vi "Marvin.vi"() -> ()   [LabVIEW 2017]
uses:
  PCAN_Driver/ControlCAN.llb/CAN Channel.ctl
  PCAN_Driver/ControlCAN.llb/DevType.ctl
  PCAN_Driver/ControlCAN.llb/VCI_INIT_CONFIG.ctl
  PCAN_Driver/ControlCAN.llb/InitFlag.ctl
  PCAN_Driver/ControlCAN.llb/Fliter.ctl
  PCAN_Driver/ControlCAN.llb/Mode.ctl
  <vilib>/Utility/miscctls.llb/LVMinMaxIncTypeDef.ctl
  PCAN_Driver/ControlCAN.llb/VCI_CAN_OBJ.ctl
  PCAN_Driver/ControlCAN.lvlib
panel:
  in  "Help Button":bool
  in  "Clear Monitor":bool
  out "Array":u64[][](array[numeric]) format="%016x"
  out "Waveform Chart":dbl[](graph)
  out "Ambient Over temp":bool
  out "Ambient Sensor temp":bool
  out "Ambient Temperature":dbl
  in  "Motor Over Temp":bool
  in  "Speed control":bool
  out "Unit Adress":string
  in  "Serial Send":bool
  in  "Index":u16(ring) items=["1"=1, "2"=2, "3"=3]
  out "read buffer":string
  in  "SetGet":enum16{"Get", "Set"}(ring)
  in  "Function":T1(ring)
  in  "Value":dbl
  in  "Value 1/2":enum16{"1", "2"}(ring)
  out "Msg Count":u32
  in  "Param to Set":u16(ring) items=["EBAY 5F"=95, "AHU 3F"=63, "AHU 2F"=47]
  out "Unit Adress":u8
  out "Horizontal Progress Bar":i32(slide) min=0 max=48 scale=0.0..50.0
  in  "Set Param.":bool
  in  "Serial Monitor":bool caption="Graph Button"
  in  "Serial Com":bool
  in  "VISA resource name":refnum<visa-resource-name>="COM6"
  out "Serial Status":bool
  in  "Graph Button":bool
  in  "Refresh Button":bool
  out "Data Send":u64 format="%016x"
  in  "Motor Speed RPM":u16
  out "Under voltage/Over voltage":bool
  out "Speed error":bool
  out "Derated drive temp":bool
  out "Motor Over temperature":bool
  out "Commutation err":bool
  out "Motor Sensor temp Fauilre":bool
  out "Drive Over temperature":bool
  out "Drive Sensor temp Failure":bool
  out "Motor Phase Current RMS":dbl
  out "ECS State":u16
  out "Motor Speed RPM":dbl
  out "Motor Stator Temp.":dbl
  out "Power transistor Heat sink Temp.":dbl
  out "DC Current":dbl
  out "DC Voltage":dbl
  in  "Can Send":bool
  in  "Stop":bool
  out "Config_CANAT":T8 {"DevType" items=["USB-CAN"=3, "USB-CAN2"=4]; "CanIndex" items=["通道1", "通道2"]; "VCI_INIT_CONFIG"."Fliter" items=["接收所有类型"=3, "只接收标准帧"=4, "只接收扩展帧"=7]; "VCI_INIT_CONFIG"."Mode" items=["正常工作", "自测模式（环回）", "仅侦听模式"]; "VCI_INIT_CONFIG"."InitFlag" items=["使用Flash参数", "使用界面设置参数"]}
  in  "Channel 2":T3 caption="Channel" items=["Channel 1", "Channel 2"]
  out "CAN Status":bool
  # "ver 1.3"
  # "Marvin"
  # "REDLER TECHNOLOGIES LTD"
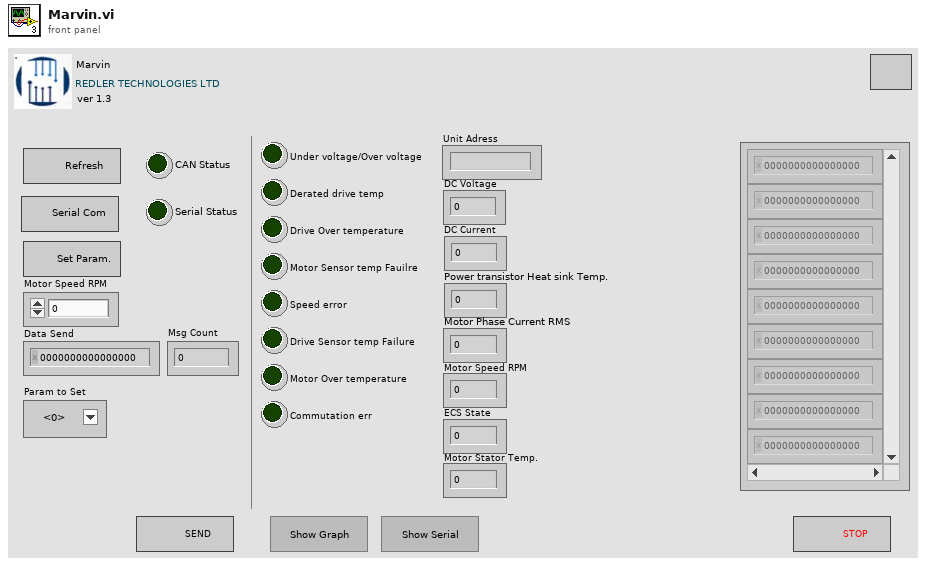
[diagram p1: front panel]
types:
  T1 = enum16{"Enable Conf. EP=1", "Serial Number", "Temperature", "Unit Adress", "Calibration", "Velocity", "Version"}
  T2 = typedef "ControlCAN.lvlib/DevType.ctl" = u32
  T3 = typedef "ControlCAN.lvlib/CAN Channel.ctl" = u32
  T4 = typedef "ControlCAN.lvlib/VCI_INIT_CONFIG.ctl" = cluster{"AccCode":u32, "AccMask":u32, "InitFlag":T5, "Fliter":T6, "Timing0":u8, "Timing1":u8, "Mode":T7}
  T5 = typedef "ControlCAN.lvlib/InitFlag.ctl" = u32
  T6 = typedef "ControlCAN.lvlib/Fliter.ctl" = u8
  T7 = typedef "ControlCAN.lvlib/Mode.ctl" = u8
  T8 = cluster{"DevType":T2, "DevIndex":u32, "CanIndex":T3, "VCI_INIT_CONFIG":T4}
  T9 = cluster{"ID":u32, "MSGTYPE":u8, "LEN":u8, "aDATA":u8[]}[]
  T10 = cluster{"ID":u32, "MSGTYPE":u8, "LEN":u8, "aDATA":u8[]}
  T11 = enum8{"Enabled", "Disabled", "Disabled and Grayed Out"}
  T12 = typedef "LVMinMaxIncTypeDef.ctl" = cluster{"Minimum":dbl, "Maximum":dbl, "Increment":dbl}
  T13 = enum32{"Invalid", "Standard", "Closed", "Hidden", "Minimized", "Maximized"}
  T14 = typedef "ControlCAN.lvlib/VCI_CAN_OBJ.ctl" = cluster{"ID":u32, "TimeStamp":u32, "TimeFlag":u8, "SendType":u8, "RemoteFlag":u8, "ExternFlag":u8, "DataLen":u8, "Data":u8[], "Reserved":u8[]}
  T15 = cluster{"Type":enum16{"接收", "发送"}, "Channel":T3, "Time":timestamp, "VCI_CAN_OBJ":T14}[]
  T16 = cluster{"Type":enum16{"接收", "发送"}, "Channel":T3, "Time":timestamp, "VCI_CAN_OBJ":T14}
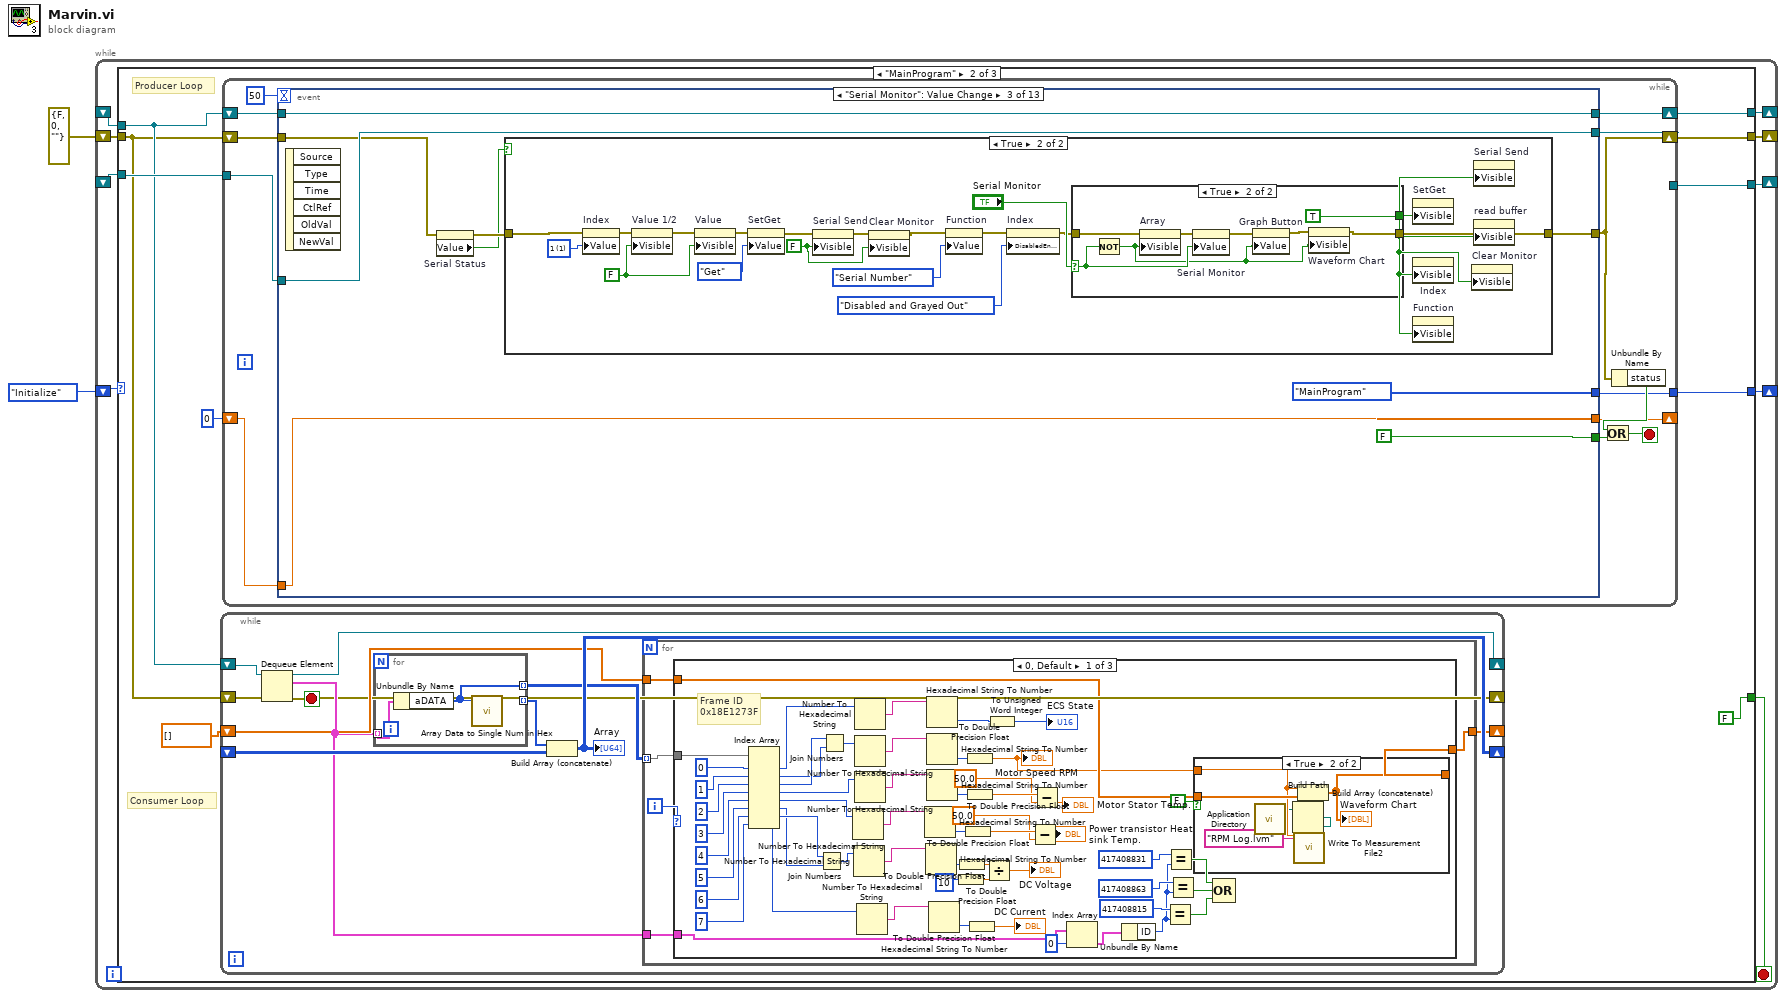
[diagram p0: block diagram]
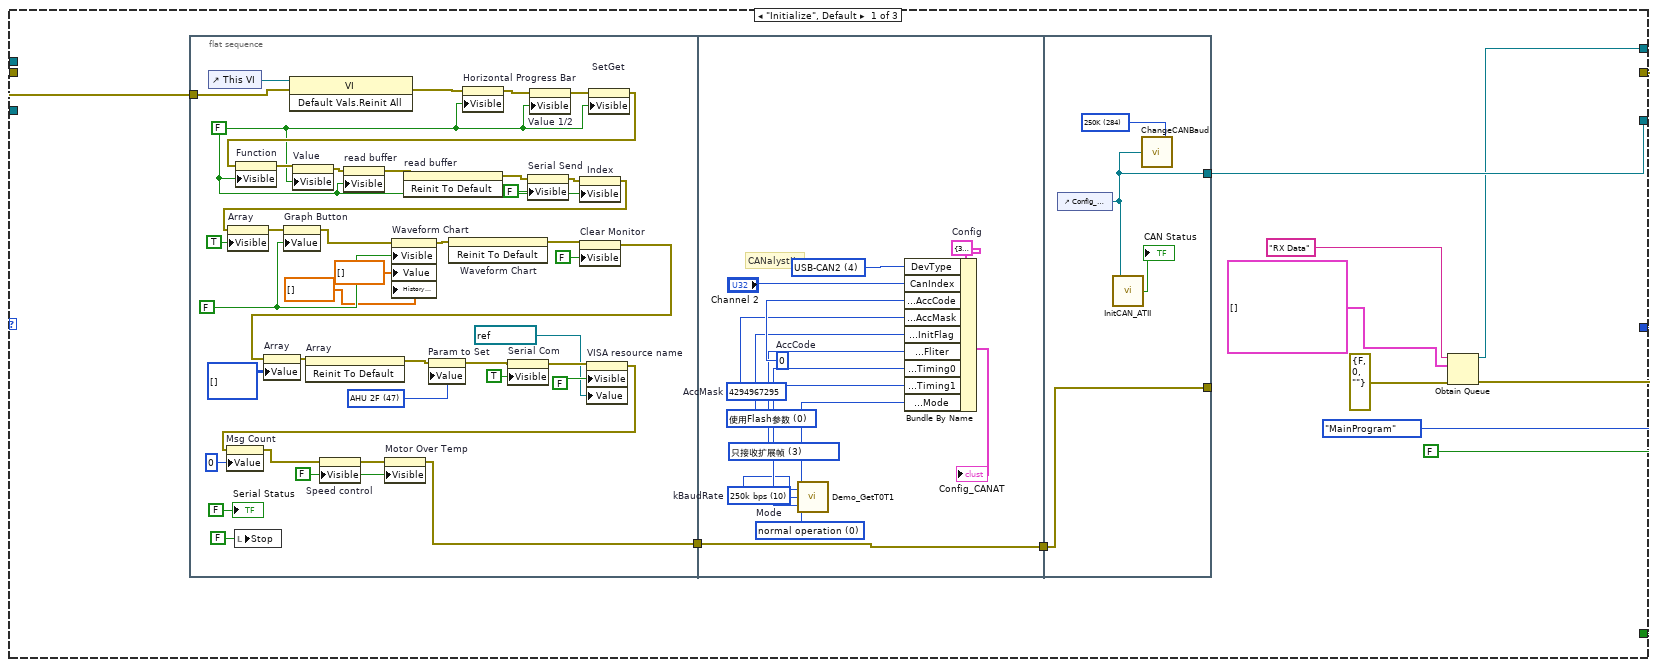
[diagram p2: hidden frame]
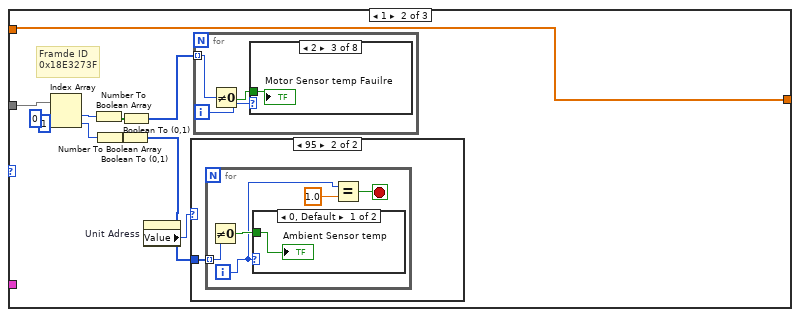
[diagram p4: hidden frame]
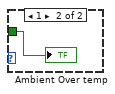
[diagram p6: hidden frame]
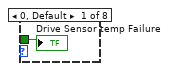
[diagram p7: hidden frame]
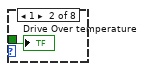
[diagram p8: hidden frame]
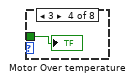
[diagram p9: hidden frame]
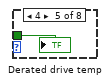
[diagram p10: hidden frame]
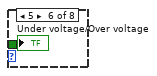
[diagram p11: hidden frame]
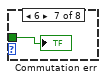
[diagram p12: hidden frame]
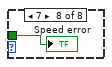
[diagram p13: hidden frame]
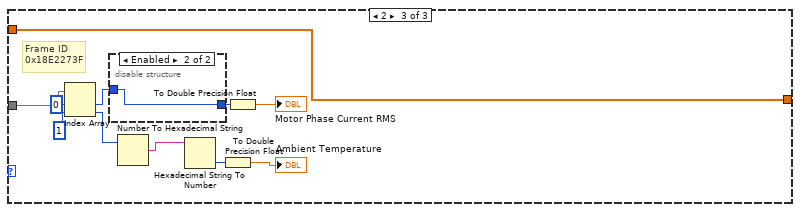
[diagram p14: hidden frame]
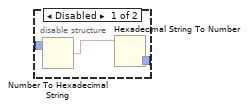
[diagram p15: hidden frame]
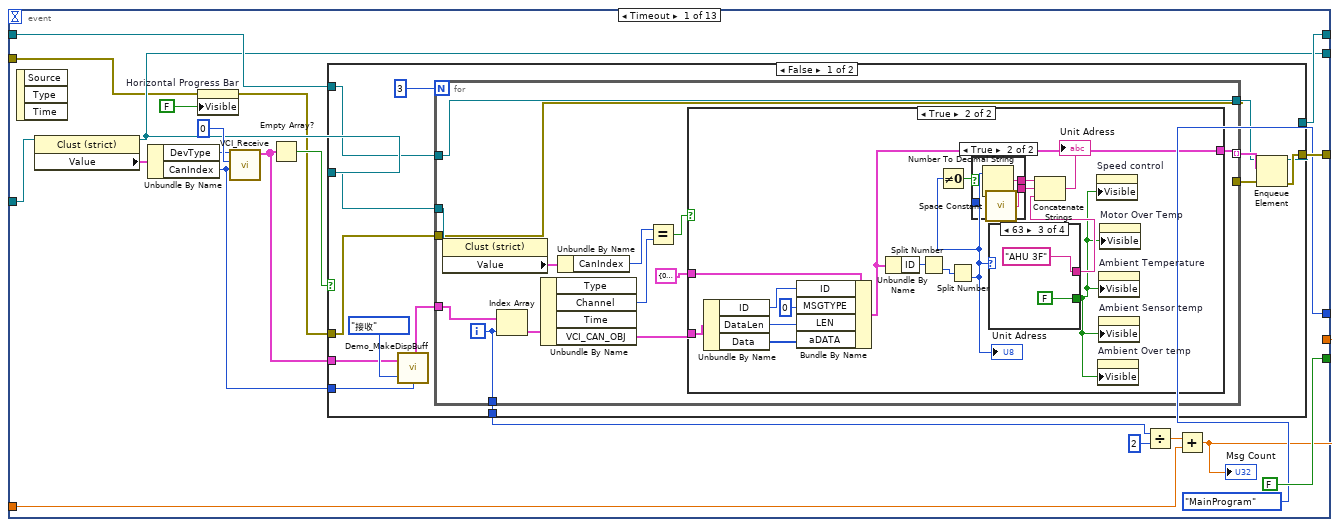
[diagram p16: hidden frame]
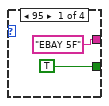
[diagram p19: hidden frame]
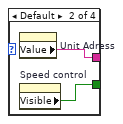
[diagram p20: hidden frame]
diagram:
  n1 = while {
    shift-right: [w6] -> _
    shift-left: enum16{"Stop", "MainProgram", "Initialize"}."Initialize" -> [w11]
    shift-right: [w10] -> _
    shift-left: _ -> [w9]
    shift-right: [w8] -> _
    shift-left: _ -> [w5]
    shift-right: [w7] -> _
    shift-left: errorcluster {"status"=FALSE, "code"=0, "source"=""} ("error out") -> [w4]
    stop <- w3 stop-if-true
    n2 = case shown="\"MainProgram\"" w11 {
      tunnel: [w22 w87 w865] -> w10
      tunnel: w9 -> [_ w90 w865]
      tunnel: [w18 w89 w866] -> w8
      tunnel: [w17 w88 w867] -> w7
      tunnel: [enum16{"Stop", "MainProgram", "Initialize"}."MainProgram" w86 enum16{"Stop", "MainProgram", "Initialize"}."Stop"] -> w6
      tunnel: w5 -> [_ w85 w866]
      tunnel: w4 -> [w15 w84 w868]
      tunnel: [FALSE ("Stop") FALSE ("Stop") w864] -> w3
      frame "Initialize", Default {
        n3 = flat-sequence {
          tunnel: w15 -> [w36]
          tunnel: [w32] -> w13
          tunnel: [w64] -> w14
          tunnel: w13 -> [w64]
          tunnel: [w78] -> w22
          tunnel: w14 -> [w77]
          tunnel: [w77] -> _
          frame #0 {
            w31 = FALSE ("Visible")
            w49 = u16 47 items=["EBAY 5F"=95, "AHU 3F"=63, "AHU 2F"=47] ("Param to Set")
            w26 = FALSE ("Visible")
            w55 = FALSE ("Graph Button")
            n4 = control-ref of="This VI"() -> (w63:refnum<vi>)
            n5 = local write "Stop"(FALSE ("Stop")) -> ()
            n6 = invoke class="VI" method="Default Vals.Reinit All"(reference=w63, error in=w36) -> (error out=w35:errorcluster)  [unwired: 1 in, 2 out]
            n7 = property on="Horizontal Progress Bar" class="Slide (strict)"(error in=w35, "Visible"=w26) -> (error out=w47:errorcluster)  [unwired: 1 in, 1 out]
            n8 = property on="Value 1/2" class="Enum (strict)"(error in=w47, "Visible"=w26) -> (error out=w46:errorcluster)  [unwired: 1 in, 1 out]
            n9 = property on="SetGet" class="Enum (strict)"(error in=w46, "Visible"=w26) -> (error out=w45:errorcluster)  [unwired: 1 in, 1 out]
            n10 = property on="Function" class="Enum (strict)"(error in=w45, "Visible"=w26) -> (error out=w44:errorcluster)  [unwired: 1 in, 1 out]
            n11 = property on="Value" class="DigNum (strict)"(error in=w44, "Visible"=w26) -> (error out=w43:errorcluster)  [unwired: 1 in, 1 out]
            n12 = property on="read buffer" class="Str"(error in=w43, "Visible"=w26) -> (error out=w28:errorcluster)  [unwired: 1 in, 1 out]
            n13 = invoke on="read buffer" class="Str" method="Reinit To Default"(error in=w28) -> (error out=w27:errorcluster)  [unwired: 2 in, 2 out]
            n14 = property on="Serial Send" class="Bool"(error in=w27, "Visible"=FALSE) -> (error out=w42:errorcluster)  [unwired: 1 in, 1 out]
            n15 = property on="Index" class="Ring (strict)"(error in=w42, "Visible"=w26) -> (error out=w41:errorcluster)  [unwired: 1 in, 1 out]
            n16 = property on="Array" class="Arr (strict)"(error in=w41, "Visible"=TRUE) -> (error out=w40:errorcluster)  [unwired: 1 in, 1 out]
            n17 = property on="Graph Button" class="Bool (strict)"(error in=w40, "Value"=w55) -> (error out=w39:errorcluster)  [unwired: 1 in, 1 out]
            n18 = property on="Waveform Chart" class="WFChart (strict)"(error in=w39, "Visible"=w55, "Value"=dbl[] [] ("Waveform Chart"), "History Data"=dbl[] []) -> (error out=w58:errorcluster)  [unwired: 1 in, 1 out]
            n19 = invoke on="Waveform Chart" class="WFChart (strict)" method="Reinit To Default"(error in=w58) -> (error out=w25:errorcluster)  [unwired: 2 in, 2 out]
            n20 = property on="Clear Monitor" class="Bool"(error in=w25, "Visible"=FALSE) -> (error out=w24:errorcluster)  [unwired: 1 in, 1 out]
            n21 = property on="Array" class="Arr (strict)"(error in=w24, "Value"=u64[][] [] ("Array")) -> (error out=w30:errorcluster)  [unwired: 1 in, 1 out]
            n22 = invoke on="Array" class="Arr (strict)" method="Reinit To Default"(error in=w30) -> (error out=w29:errorcluster)  [unwired: 2 in, 2 out]
            n23 = property on="Param to Set" class="Ring (strict)"(error in=w29, "Value"=w49) -> (error out=w38:errorcluster)  [unwired: 1 in, 1 out]
            n24 = property on="Serial Com" class="Bool"(error in=w38, "Visible"=TRUE) -> (error out=w60:errorcluster)  [unwired: 1 in, 1 out]
            n25 = property on="VISA resource name" class="VISAName"(error in=w60, "Visible"=FALSE, "Value"=refnum<visa-resource-name> "COM1" ("VISA resource name")) -> (error out=w37:errorcluster)  [unwired: 1 in, 1 out]
            n26 = property on="Msg Count" class="DigNum (strict)"(error in=w37, "Value"=u32 0 ("Msg Count")) -> (error out=w34:errorcluster)  [unwired: 1 in, 1 out]
            n27 = property on="Speed control" class="Bool (strict)"(error in=w34, "Visible"=w31) -> (error out=w33:errorcluster)  [unwired: 1 in, 1 out]
            n28 = property on="Motor Over Temp" class="Bool (strict)"(error in=w33, "Visible"=w31) -> (error out=w32:errorcluster)  [unwired: 1 in, 1 out]
            "Serial Status" <- FALSE ("Serial Status")
          }
          frame #1 {
            w68 = u32 4294967295  # AccMask
            w67 = T5 0 items=["使用Flash参数", "使用界面设置参数"] ("InitFlag")
            w65 = T7 0 items=["normal operation", "Listen-only mode", "test mode"]  # Mode
            w66 = T6 3 items=["接收所有类型"=1, "只接收标准帧"=2, "只接收扩展帧"=3] ("Fliter")
            w72 = u8 10 items=["5k bps"=1, "10k bps"=2, "20k bps"=3, "40k bps"=4, "50k bps"=5, "80k bps"=6, "100k bps"=7, "125k bps"=8, "200k bps"=9, "250k bps"=10, "400k bps"=11, "500k bps"=12, "666k bps"=13, "800k bps"=14, "1000k bps"=15, "33.33k bps"=16, "66.66k bps"=17, "83.33k bps"=18]  # kBaudRate
            w69 = u32 0  # AccCode
            w70 = T2 4 items=["USB-CAN"=3, "USB-CAN2"=4] ("DevType")
            w71 = T8 {"DevType"=3, "DevIndex"=0, "CanIndex"=0, "VCI_INIT_CONFIG"={"AccCode"=0, "AccMask"=0, "InitFlag"=1, "Fliter"=7, "Timing0"=0, "Timing1"=0, "Mode"=0}}  # Config
            # "CANalystII"
            n29 = call "Demo_GetT0T1.vi"("kBaudRate"=w72) -> ("Timing0"=w74:u8, "Timing1"=w75:u8)
            n30 = Bundle By Name(cluster=w71, "DevType"=w70, "CanIndex"="Channel 2", "VCI_INIT_CONFIG.AccCode"=w69, "VCI_INIT_CONFIG.AccMask"=w68, "VCI_INIT_CONFIG.InitFlag"=w67, "VCI_INIT_CONFIG.Fliter"=w66, "VCI_INIT_CONFIG.Timing0"=w74, "VCI_INIT_CONFIG.Timing1"=w75, "VCI_INIT_CONFIG.Mode"=w65) -> (→"Config_CANAT":T8)
          }
          frame #2 {
            w79 = u16 284 items=["1M"=20, "500K"=28, "250K"=284, "125K"=796, "100K"=17199, "50K"=18223, "20K"=21295, "10K"=26415, "5K"=32639] ("baud in")
            n31 = control-ref of="Config_CANAT"() -> (w78:refnum<vi>)
            n32 = call "InitCAN_ATII.vi"("Config"=w78) -> ("Sts"=→"CAN Status":bool)
            n33 = call "ChangeCANBaud.vi"("baud in"=w79, "reference"=w78) -> ()
          }
        }
        n34 = Obtain Queue(name (unnamed)="RX Data", element data type=T9 [], error in (no error)=errorcluster {"status"=FALSE, "code"=0, "source"=""}) -> (queue out=w18:refnum<queue>, error out=w17:errorcluster)  [unwired: 2 in, 1 out]
      }
      frame "MainProgram" {
        # "Consumer Loop"
        # "Producer Loop"
        n35 = while {
          shift-right: [w99] -> _
          shift-left: w85 -> [w101]
          shift-right: [w97] -> _
          shift-left: _ -> [w98]
          shift-right: [w94] -> _
          shift-left: dbl[] [] -> [w93]
          shift-right: [w91] -> _
          shift-left: w84 -> [w91]
          stop <- w100 stop-if-true
          n36 = Dequeue Element(queue=w101, error in (no error)=w91) -> (queue out=w99:refnum<queue>, element=w92:T9, error out=w100:errorcluster)  [unwired: 1 in, 1 out]
          n37 = for {
            tunnel: [w218] -> w96 mode=indexing
            tunnel: w92 -> [w217] mode=indexing
            tunnel: [w216] -> w95 mode=indexing
            n38 = Unbundle By Name(w217) -> ("aDATA"=w216:u8[])
            n39 = call "Array Data to Single Num in Hex.vi"("aDATA"=w216) -> ("Numeric"=w218:u64)  [unwired: 10 in]
          }
          n40 = Build Array (concatenate)(w96, w98) -> (w97:u64[][])
          "Array" <- w97
          n41 = for {
            tunnel: w95 -> [w106] mode=indexing
            tunnel: [w104] -> w94
            tunnel: w93 -> [w103]
            tunnel: w92 -> [w102]
            i -> [w105]
            n42 = case shown="0, Default" w105 {
              tunnel: w106 -> [w145 w181 w211]
              tunnel: [w119 w176 w206] -> w104
              tunnel: w103 -> [w120 w176 w206]
              tunnel: w102 -> [w118 _ _]
              frame 0, Default {
                # "Frame ID\n0x18E1273F"
                n43 = Index Array(array=w145, index #1=0 ("index"), index #2=1 ("index"), index #3=2 ("index"), index #4=3 ("index"), index #5=4 ("index"), index #6=5 ("index"), index #7=6 ("index"), index #8=7 ("index")) -> (element #1=w129:u8, element #2=w131:u8, element #3=w132:u8, element #4=w136:u8, element #5=w139:u8, element #6=w143:u8, element #7=w144:u8, element #8=w142:u8)
                n44 = Join Numbers(hi=w144, lo=w143) -> ((hi.lo)=w163:u16)
                n45 = Join Numbers(hi=w132, lo=w131) -> ((hi.lo)=w133:u16)
                n46 = Number To Hexadecimal String(2:w139) -> (0:w140:string)  [unwired: 1 in]
                n47 = Number To Hexadecimal String(2:w163) -> (0:w162:string)  [unwired: 1 in]
                n48 = Number To Hexadecimal String(2:w129) -> (0:w130:string)  [unwired: 1 in]
                n49 = Number To Hexadecimal String(2:w133) -> (0:w134:string)  [unwired: 1 in]
                n50 = Number To Hexadecimal String(2:w136) -> (0:w137:string)  [unwired: 1 in]
                n51 = Number To Hexadecimal String(2:w142) -> (0:w156:string)  [unwired: 1 in]
                n52 = Hexadecimal String To Number(string=w140) -> (number=w141:u32)  [unwired: 2 in, 1 out]
                n53 = Hexadecimal String To Number(string=w162) -> (number=w161:u32)  [unwired: 2 in, 1 out]
                n54 = Hexadecimal String To Number(string=w130) -> (number=w127:u32)  [unwired: 2 in, 1 out]
                n55 = Hexadecimal String To Number(string=w134) -> (number=w135:u32)  [unwired: 2 in, 1 out]
                n56 = Hexadecimal String To Number(string=w137) -> (number=w138:u32)  [unwired: 2 in, 1 out]
                n57 = Hexadecimal String To Number(string=w156) -> (number=w155:u32)  [unwired: 2 in, 1 out]
                n58 = To Double Precision Float(number=u32 10 ("y")) -> (double precision float=w159:dbl)
                n59 = To Double Precision Float(number=w161) -> (double precision float=w158:dbl)
                n60 = To Double Precision Float(number=w141) -> (double precision float=w122:dbl)
                n61 = To Double Precision Float(number=w135) -> (double precision float=w115:dbl)
                "Motor Speed RPM" <- w115
                n62 = To Double Precision Float(number=w138) -> (double precision float=w124:dbl)
                n63 = To Double Precision Float(number=w155) -> (double precision float=→"DC Current":dbl)
                n64 = Divide(x=w158, y=w159) -> (x/y=→"DC Voltage":dbl)
                n65 = To Unsigned Word Integer(number=w127) -> (unsigned 16bit integer=→"ECS State":u16)
                n66 = Subtract(x=w122, y=50.0 ("x")) -> (x-y=→"Power transistor Heat sink Temp.":dbl)
                n67 = Subtract(x=w124, y=50.0 ("x")) -> (x-y=→"Motor Stator Temp.":dbl)
                n68 = Index Array(array=w118, index=0) -> (element=w116:T10)
                n69 = Unbundle By Name(w116) -> ("ID"=w108:u32)
                n70 = Equal?(x=u32 417408815, y=w108) -> (x = y?=w109:bool)
                n71 = Equal?(x=u32 417408831, y=w108) -> (x = y?=w111:bool)
                n72 = Equal?(x=u32 417408863, y=w108) -> (x = y?=w110:bool)
                n73 = case shown="True" FALSE {
                  tunnel: w120 -> [w164 w170]
                  tunnel: [w164 w169] -> w119
                  tunnel: w115 -> [_ w168]
                  frame False {
                  }
                  frame True {
                    n74 = call <vilib>:"Application Directory.vi"() -> ("Application Directory"=w166:path)
                    n75 = Build Path(base path=w166, name or relative path="RPM Log.lvm") -> (appended path=w167:path)
                    n76 = call "Write To Measurement File2"("Signals"=w168, "Filename"=w167) -> ()  [unwired: 15 in, 3 out]
                    n77 = Build Array (concatenate)(w168, w170) -> (w169:dbl[])
                    "Waveform Chart" <- w169
                  }
                }
                n78 = Compound Arithmetic op=OR(w111, w110, w109) -> ()  [unwired: 1 out]
              }
              frame 1 {
                # "Framde ID\n0x18E3273F"
                n79 = Index Array(array=w181, index #1=0 ("index"), index #2=1 ("index")) -> (element #1=w179:u8, element #2=w173:u8)
                n80 = Number To Boolean Array(number=w179) -> (Boolean array=w178:bool[])
                n81 = Number To Boolean Array(number=w173) -> (Boolean array=w175:bool[])
                n82 = Boolean To (0,1)(Boolean=w175) -> (0, 1=w172:i16[])
                n83 = Boolean To (0,1)(Boolean=w178) -> (0, 1=w177:i16[])
                n84 = property on="Unit Adress" class="DigNum (strict)"() -> ("Value"=w171:u8)  [unwired: 2 in, 2 out]
                n85 = case shown="95" w171 {
                  tunnel: w172 -> [_ w182]
                  frame 0, Default {
                  }
                  frame 95 {
                    n86 = for {
                      tunnel: w182 -> [w187] mode=indexing
                      i -> [w183]
                      stop <- w185 stop-if-true
                      n87 = Not Equal To 0?(x=w187) -> (x != 0?=w186:bool)
                      n88 = case shown="0, Default" w183 {
                        tunnel: w186 -> [w188 w189]
                        frame 0, Default {
                          "Ambient Sensor temp" <- w188
                        }
                        frame 1 {
                          "Ambient Over temp" <- w189
                        }
                      }
                      n89 = Equal?(x=w183, y=1.0) -> (x = y?=w185:bool)
                    }
                  }
                }
                n90 = for {
                  tunnel: w177 -> [w191] mode=indexing
                  i -> [w192]
                  n91 = Not Equal To 0?(x=w191) -> (x != 0?=w190:bool)
                  n92 = case shown="2" w192 {
                    tunnel: w190 -> [w193 w194 w195 w196 w197 w198 w199 w200]
                    frame 0, Default {
                      "Drive Sensor temp Failure" <- w193
                    }
                    frame 1 {
                      "Drive Over temperature" <- w194
                    }
                    frame 2 {
                      "Motor Sensor temp Fauilre" <- w195
                    }
                    frame 3 {
                      "Motor Over temperature" <- w196
                    }
                    frame 4 {
                      "Derated drive temp" <- w197
                    }
                    frame 5 {
                      "Under voltage/Over voltage" <- w198
                    }
                    frame 6 {
                      "Commutation err" <- w199
                    }
                    frame 7 {
                      "Speed error" <- w200
                    }
                  }
                }
              }
              frame 2 {
                # "Frame ID\n0x18E2273F"
                n93 = Index Array(array=w211, index #1=0 ("index"), index #2=1 ("index")) -> (element #1=w208:u8, element #2=w204:u8)
                n94 = disable-structure shown="Enabled" {
                  disable-tunnel: [w214 w215] -> w209
                  disable-tunnel: w208 -> [w213 w215]
                  frame Disabled {
                    n95 = Number To Hexadecimal String(2:w213) -> (0:w212:string)  [unwired: 1 in]
                    n96 = Hexadecimal String To Number(string=w212) -> (number=w214:u32)  [unwired: 2 in, 1 out]
                  }
                  frame Enabled {
                  }
                }
                n97 = Number To Hexadecimal String(2:w204) -> (0:w202:string)  [unwired: 1 in]
                n98 = Hexadecimal String To Number(string=w202) -> (number=w203:u32)  [unwired: 2 in, 1 out]
                n99 = To Double Precision Float(number=w203) -> (double precision float=→"Ambient Temperature":dbl)
                n100 = To Double Precision Float(number=w209) -> (double precision float=→"Motor Phase Current RMS":dbl)
              }
            }
          }
        }
        n101 = while {
          shift-right: [w225] -> w88
          shift-left: w84 -> [w227]
          shift-right: [w226] -> w89
          shift-left: w85 -> [w228]
          tunnel: w90 -> [w229]
          tunnel: [w222] -> w87
          tunnel: [w221] -> w86
          shift-right: [w219] -> _
          shift-left: 0 -> [w220]
          stop <- w230 stop-if-true
          n102 = event shown="[2] \"Serial Monitor\": Value Change" {
            selector: _ -> [_ _ _ _ _ _ _ _ _ _ _ _ _]
            dyn-events: _ -> [_ _ _ _ _ _ _ _ _ _ _ _ _]
            timeout: 50 -> [_ _ _ _ _ _ _ _ _ _ _ _ _]
            tunnel: w229 -> [w249 w321 w331 w391 w574 w620 w717 w737 w805 w825 w840 w855 w861]
            tunnel: w228 -> [w246 w322 w334 w392 w575 w619 w718 w758 w806 w824 w841 w852 w858]
            tunnel: w227 -> [w238 w320 w329 w386 w577 w611 w710 w757 w798 w820 w833 w851 w859]
            tunnel: [w244 w322 w334 w392 w575 w619 w718 w758 w806 w824 w841 w850 w858] -> w226
            tunnel: [w243 w312 w330 w383 w576 w615 w707 w757 w786 w817 w830 w848 w857] -> w225
            tunnel: [FALSE ("Stop") FALSE ("Stop") FALSE ("Stop") FALSE ("Stop") FALSE ("Stop") FALSE ("Stop") FALSE ("Stop") FALSE ("Stop") FALSE ("Stop") FALSE ("Stop") FALSE ("Stop") TRUE ("Stop") TRUE ("Stop")] -> w223
            tunnel: [w242 w321 w331 w391 w574 w620 w717 w737 w805 w825 w840 w855 w861] -> w222
            tunnel: [enum16{"Stop", "MainProgram", "Initialize"}."MainProgram" enum16{"Stop", "MainProgram", "Initialize"}."MainProgram" enum16{"Stop", "MainProgram", "Initialize"}."MainProgram" enum16{"Stop", "MainProgram", "Initialize"}."MainProgram" enum16{"Stop", "MainProgram", "Initialize"}."MainProgram" enum16{"Stop", "MainProgram", "Initialize"}."MainProgram" enum16{"Stop", "MainProgram", "Initialize"}."MainProgram" enum16{"Stop", "MainProgram", "Initialize"}."MainProgram" enum16{"Stop", "MainProgram", "Initialize"}."MainProgram" enum16{"Stop", "MainProgram", "Initialize"}."MainProgram" enum16{"Stop", "MainProgram", "Initialize"}."MainProgram" enum16{"Stop", "MainProgram", "Initialize"}."Stop" enum16{"Stop", "MainProgram", "Initialize"}."Initialize"] -> w221
            tunnel: w220 -> [w237 w325 w327 w379 w573 w609 w721 w722 w796 w816 w827 w847 w856]
            tunnel: [w236 w325 w327 w379 w573 w609 w721 w722 w796 w816 w827 w847 w856] -> w219
            event Timeout {
              n103 = event-data() -> ()  [unwired: 1 in, 3 out]
              n104 = property class="Clust (strict)"(reference=w249) -> (reference out=w242:refnum<vi>, "Value"=w250:T8)  [unwired: 1 in, 1 out]
              n105 = Unbundle By Name(w250) -> ("DevType"=w251:T2, "CanIndex"=w247:T3)
              n106 = property on="Horizontal Progress Bar" class="Slide (strict)"(error in=w238, "Visible"=FALSE) -> (error out=w232:errorcluster)  [unwired: 1 in, 1 out]
              n107 = call "VCI_Receive.vi"("CANIndex"=w247, "DevIndex"=u32 0, "DevType"=w251) -> ("Recieve"=w245:T14[])  [unwired: 3 in, 5 out]
              n108 = Empty Array?(array=w245) -> (empty?=w248:bool)
              n109 = case shown="False" w248 {
                tunnel: w247 -> [w264 _]
                tunnel: w242 -> [w262 _]
                tunnel: w246 -> [w261 w310]
                tunnel: w232 -> [w260 w309]
                tunnel: w245 -> [w265 _]
                tunnel: [w255 w309] -> w243
                tunnel: [w254 w310] -> w244
                tunnel: [w253 0] -> w233
                frame False {
                  n110 = call "Demo_MakeDispBuff.vi"("Channel"=w264, "Type"=enum16{"接收", "发送"}."接收", "OBJs"=w265) -> ("Buffer"=w263:T15)
                  n111 = for {
                    N: 3 -> [_]
                    tunnel: w263 -> [w279]
                    tunnel: w262 -> [w278]
                    tunnel: w261 -> [w269]
                    tunnel: w260 -> [w268]
                    tunnel: [w271] -> w258 mode=indexing
                    tunnel: [w269] -> w257
                    tunnel: [w268] -> w256
                    tunnel: [w267] -> w253
                    i -> [w267]
                    n112 = property class="Clust (strict)"(reference=w278) -> ("Value"=w276:T8)  [unwired: 1 in, 2 out]
                    n113 = Index Array(array=w279, index=w267) -> (element=w272:T16)
                    n114 = Unbundle By Name(w272) -> ("Channel"=w274:T3, "VCI_CAN_OBJ"=w277:T14)  [unwired: 2 out]
                    n115 = Unbundle By Name(w276) -> ("CanIndex"=w275:T3)
                    n116 = Equal?(x=w275, y=w274) -> (x = y?=w273:bool)
                    n117 = case shown="True" w273 {
                      tunnel: w277 -> [_ w296]
                      tunnel: [w280 w292] -> w271
                      tunnel: T10 {"ID"=0, "MSGTYPE"=0, "LEN"=0, "aDATA"=[]} ("Msg") -> [w280 w291]
                      frame False {
                      }
                      frame True {
                        n118 = Unbundle By Name(w296) -> ("ID"=w290:u32, "DataLen"=w295:u8, "Data"=w293:u8[])
                        n119 = Bundle By Name(cluster=w291, "ID"=w290, "MSGTYPE"=u8 0, "LEN"=w295, "aDATA"=w293) -> (w292:T10)
                        n120 = Unbundle By Name(w292) -> ("ID"=w288:u32)
                        n121 = Split Number(x=w288) -> (lo(x)=w289:u16)  [unwired: 1 out]
                        n122 = Split Number(x=w289) -> (lo(x)=w281:u8)  [unwired: 1 out]
                        "Unit Adress" <- w281
                        n123 = Not Equal To 0?(x=w281) -> (x != 0?=w282:bool)
                        n124 = case shown="True" w282 {
                          tunnel: w281 -> [_ w299]
                          tunnel: [_ w298] -> w287
                          tunnel: [_ w297] -> w284
                          frame False {
                          }
                          frame True {
                            n125 = Number To Decimal String(number=w299) -> (decimal integer string=w298:string)  [unwired: 1 in]
                            n126 = call <vilib>:"Space Constant.vi"() -> ("String"=w297:string)
                          }
                        }
                        n127 = case shown="63" w281 {
                          tunnel: ["EBAY 5F" w302 "AHU 3F" "AHU 2F"] -> w286
                          tunnel: [TRUE w303 FALSE FALSE] -> w283
                          frame 95 {
                          }
                          frame Default {
                            n128 = property on="Unit Adress" class="Str"() -> ("Value"=w302:string)  [unwired: 2 in, 2 out]
                            n129 = property on="Speed control" class="Bool (strict)"() -> ("Visible"=w303:bool)  [unwired: 2 in, 2 out]
                          }
                          frame 63 {
                          }
                          frame 47 {
                          }
                        }
                        n130 = Concatenate Strings(w287, w284, w286) -> (→"Unit Adress":string)
                        n131 = property on="Speed control" class="Bool (strict)"("Visible"=w283) -> ()  [unwired: 2 in, 2 out]
                        n132 = property on="Ambient Over temp" class="Bool (strict)"("Visible"=w283) -> ()  [unwired: 2 in, 2 out]
                        n133 = property on="Ambient Temperature" class="DigNum (strict)"("Visible"=w283) -> ()  [unwired: 2 in, 2 out]
                        n134 = property on="Ambient Sensor temp" class="Bool (strict)"("Visible"=w283) -> ()  [unwired: 2 in, 2 out]
                        n135 = property on="Motor Over Temp" class="Bool (strict)"("Visible"=w283) -> ()  [unwired: 2 in, 2 out]
                      }
                    }
                  }
                  n136 = Enqueue Element(queue=w257, element=w258, error in (no error)=w256) -> (queue out=w254:refnum<queue>, error out=w255:errorcluster)  [unwired: 2 out]
                }
                frame True {
                }
              }
              n137 = Divide(x=w233, y=u32 2) -> (x/y=w234:dbl)
              n138 = Add(x=w234, y=w237) -> (x+y=w236:dbl)
              "Msg Count" <- w236
            }
            event "Clear Monitor": Value Change {
              n139 = event-data() -> ()  [unwired: 1 in, 6 out]
              n140 = property on="VISA resource name" class="VISAName"(error in=w320) -> (error out=w319:errorcluster, "Value"=w316:refnum<visa-resource-name>)  [unwired: 1 in, 1 out]
              n141 = call "Serial.vi"("error in (no error)"=w319, "Clear Log"=TRUE, "VISA resource name"=w316) -> ("error out"=w314:errorcluster, "read buffer"=w315:string)  [unwired: 7 in]
              n142 = property on="read buffer" class="Str"(error in=w314, "Value"=w315) -> (error out=w313:errorcluster)  [unwired: 1 in, 1 out]
              n143 = call "Serial.vi"("error in (no error)"=w313, "Clear Log"=FALSE, "write buffer"="" ("read buffer"), "VISA resource name"=w316) -> ("error out"=w312:errorcluster)  [unwired: 6 in, 1 out]
            }
            event "Serial Monitor": Value Change {
              n144 = event-data() -> ()  [unwired: 1 in, 6 out]
              n145 = property on="Serial Status" class="Bool (strict)"(error in=w329) -> (error out=w328:errorcluster, "Value"=w326:bool)  [unwired: 1 in, 1 out]
              n146 = case shown="True" w326 {
                tunnel: w328 -> [w338 w351]
                tunnel: [w336 w356] -> w330
                frame False {
                  n147 = call "Display Message to User3"("error in (no error)"=w338) -> ("error out"=w337:errorcluster)  [unwired: 9 in, 1 out]
                  n148 = property on="Serial Monitor" class="Bool (strict)"(error in=w337, "Value"=FALSE ("Serial Monitor")) -> (error out=w336:errorcluster)  [unwired: 1 in, 1 out]
                }
                frame True {
                  w343 = FALSE ("Visible")
                  w353 = FALSE ("Visible")
                  w354 = u16 1 items=["1"=1, "2"=2, "3"=3] ("Index")
                  n149 = property on="Index" class="Ring (strict)"(error in=w351, "Value"=w354) -> (error out=w350:errorcluster)  [unwired: 1 in, 1 out]
                  n150 = property on="Value 1/2" class="Enum (strict)"(error in=w350, "Visible"=w353) -> (error out=w349:errorcluster)  [unwired: 1 in, 1 out]
                  n151 = property on="Value" class="DigNum (strict)"(error in=w349, "Visible"=w353) -> (error out=w348:errorcluster)  [unwired: 1 in, 1 out]
                  n152 = property on="SetGet" class="Enum (strict)"(error in=w348, "Value"=enum16{"Get", "Set"}."Get" ("SetGet")) -> (error out=w347:errorcluster)  [unwired: 1 in, 1 out]
                  n153 = property on="Serial Send" class="Bool"(error in=w347, "Visible"=w343) -> (error out=w342:errorcluster)  [unwired: 1 in, 1 out]
                  n154 = property on="Clear Monitor" class="Bool"(error in=w342, "Visible"=w343) -> (error out=w341:errorcluster)  [unwired: 1 in, 1 out]
                  n155 = property on="Function" class="Enum (strict)"(error in=w341, "Value"=T1."Serial Number" ("Function")) -> (error out=w346:errorcluster)  [unwired: 1 in, 1 out]
                  n156 = property on="Index" class="Ring (strict)"(error in=w346, "DisabledEnum"=T11."Disabled and Grayed Out" ("Disabled")) -> (error out=w344:errorcluster)  [unwired: 1 in, 1 out]
                  n157 = case shown="True" "Serial Monitor" {
                    selector: "Serial Monitor" -> [w360 w375]
                    tunnel: w344 -> [w359 w378]
                    tunnel: [w362 w372] -> w356
                    tunnel: [FALSE TRUE] -> w340
                    frame False {
                      n158 = property on="Graph Button" class="Bool (strict)"(error in=w359) -> (error out=w358:errorcluster, "Value"=w357:bool)  [unwired: 1 in, 1 out]
                      n159 = case shown="True" w357 {
                        tunnel: [w367 w370] -> w363
                        tunnel: w358 -> [w366 w369]
                        tunnel: w360 -> [w364 _]
                        frame False {
                          n160 = Not(x=w364) -> (.not. x?=w365:bool)
                          n161 = property on="Array" class="Arr (strict)"(error in=w366, "Visible"=w365) -> (error out=w367:errorcluster)  [unwired: 1 in, 1 out]
                        }
                        frame True {
                          n162 = property on="Array" class="Arr (strict)"(error in=w369, "Visible"=FALSE) -> (error out=w370:errorcluster)  [unwired: 1 in, 1 out]
                        }
                      }
                      n163 = property on="Serial Monitor" class="Bool (strict)"(error in=w363, "Value"=w360) -> (error out=w362:errorcluster)  [unwired: 1 in, 1 out]
                    }
                    frame True {
                      n164 = Not(x=w375) -> (.not. x?=w371:bool)
                      n165 = property on="Array" class="Arr (strict)"(error in=w378, "Visible"=w371) -> (error out=w377:errorcluster)  [unwired: 1 in, 1 out]
                      n166 = property on="Serial Monitor" class="Bool (strict)"(error in=w377, "Value"=w375) -> (error out=w374:errorcluster)  [unwired: 1 in, 1 out]
                      n167 = property on="Graph Button" class="Bool (strict)"(error in=w374, "Value"=w371) -> (error out=w373:errorcluster)  [unwired: 1 in, 1 out]
                      n168 = property on="Waveform Chart" class="WFChart (strict)"(error in=w373, "Visible"=w371) -> (error out=w372:errorcluster)  [unwired: 1 in, 1 out]
                    }
                  }
                  n169 = property on="SetGet" class="Enum (strict)"("Visible"=w340) -> ()  [unwired: 2 in, 2 out]
                  n170 = property on="Index" class="Ring (strict)"("Visible"=w340) -> ()  [unwired: 2 in, 2 out]
                  n171 = property on="Function" class="Enum (strict)"("Visible"=w340) -> ()  [unwired: 2 in, 2 out]
                  n172 = property on="Clear Monitor" class="Bool"("Visible"=w340) -> ()  [unwired: 2 in, 2 out]
                  n173 = property on="Serial Send" class="Bool"("Visible"=w340) -> ()  [unwired: 2 in, 2 out]
                  n174 = property on="read buffer" class="Str"("Visible"=w340) -> ()  [unwired: 2 in, 2 out]
                }
              }
            }
            event "Serial Send": Value Change {
              n175 = event-data() -> ()  [unwired: 1 in, 6 out]
              n176 = property on="read buffer" class="Str"(error in=w386) -> (error out=w385:errorcluster, "Text.Scroll Position"=w382:u32)  [unwired: 1 in, 1 out]
              n177 = property on="VISA resource name" class="VISAName"() -> ("Value"=w393:refnum<visa-resource-name>)  [unwired: 2 in, 2 out]
              n178 = case shown="\"Set\"" "SetGet" {
                tunnel: "Function" -> [w400 w479]
                tunnel: w393 -> [w406 w492]
                tunnel: w385 -> [w403 w478]
                tunnel: "Value" -> [_ w491]
                tunnel: "Value 1/2" -> [_ w489]
                tunnel: "Index" -> [w401 w486]
                tunnel: [w405 w484] -> w384
                tunnel: [w398 w482] -> w390
                frame "Get", Default {
                  w404 = FALSE ("Visible")
                  n179 = property on="Value" class="DigNum (strict)"(error in=w403, "Visible"=w404) -> (error out=w402:errorcluster)  [unwired: 1 in, 1 out]
                  n180 = property on="Value 1/2" class="Enum (strict)"(error in=w402, "Visible"=w404) -> (error out=w399:errorcluster)  [unwired: 1 in, 1 out]
                  n181 = case shown="\"Velocity\"" w400 {
                    tunnel: w406 -> [w410 w427 w442 w450 w456 w466]
                    tunnel: w399 -> [w408 w418 w432 w445 w454 w464]
                    tunnel: [w413 w428 w443 w451 w460 w467] -> w405
                    tunnel: [w412 w429 w441 w452 w461 w462] -> w398
                    tunnel: w401 -> [_ w422 w434 _ _ _]
                    frame "Serial Number", Default {
                      n182 = Concatenate Strings("SN" ("string"), "\r\n" ("write buffer")) -> (w411:string)
                      n183 = property on="Index" class="Ring (strict)"(error in=w408, "DisabledEnum"=T11."Disabled and Grayed Out" ("Disabled")) -> (error out=w407:errorcluster)  [unwired: 1 in, 1 out]
                      n184 = call "Serial.vi"("error in (no error)"=w407, "write buffer"=w411, "VISA resource name"=w410) -> ("error out"=w413:errorcluster, "read buffer"=w412:string)  [unwired: 7 in]
                    }
                    frame "Temperature" {
                      n185 = Number To Decimal String(number=w422) -> (decimal integer string=w421:string)  [unwired: 1 in]
                      n186 = property on="Index" class="Ring (strict)"(error in=w418, "DisabledEnum"=T11."Enabled" ("Disabled"), "Visible"=TRUE) -> (error out=w417:errorcluster)  [unwired: 1 in, 1 out]
                      n187 = Concatenate Strings("TA" ("string"), "[", w421, "]", "\r\n" ("write buffer")) -> (w423:string)
                      n188 = call "Serial.vi"("error in (no error)"=w417, "write buffer"=w423, "VISA resource name"=w427) -> ("error out"=w428:errorcluster, "read buffer"=w429:string)  [unwired: 7 in]
                    }
                    frame "Unit Adress" {
                      n189 = Number To Decimal String(number=w434) -> (decimal integer string=w440:string)  [unwired: 1 in]
                      n190 = property on="Index" class="Ring (strict)"(error in=w432, "DisabledEnum"=T11."Enabled" ("Disabled"), "Visible"=TRUE) -> (error out=w431:errorcluster)  [unwired: 1 in, 1 out]
                      n191 = Concatenate Strings("UA" ("string"), "[", w440, "]", "\r\n" ("write buffer")) -> (w435:string)
                      n192 = call "Serial.vi"("error in (no error)"=w431, "write buffer"=w435, "VISA resource name"=w442) -> ("error out"=w443:errorcluster, "read buffer"=w441:string)  [unwired: 7 in]
                    }
                    frame "Calibration" {
                      n193 = Concatenate Strings("CC" ("string"), "\r\n" ("write buffer")) -> (w448:string)
                      n194 = property on="Index" class="Ring (strict)"(error in=w445, "DisabledEnum"=T11."Disabled and Grayed Out" ("Disabled")) -> (error out=w444:errorcluster)  [unwired: 1 in, 1 out]
                      n195 = call "Serial.vi"("error in (no error)"=w444, "write buffer"=w448, "VISA resource name"=w450) -> ("error out"=w451:errorcluster, "read buffer"=w452:string)  [unwired: 7 in]
                    }
                    frame "Velocity" {
                      n196 = Concatenate Strings("VC" ("string"), "\r\n" ("write buffer")) -> (w457:string)
                      n197 = property on="Index" class="Ring (strict)"(error in=w454, "DisabledEnum"=T11."Disabled and Grayed Out" ("Disabled")) -> (error out=w453:errorcluster)  [unwired: 1 in, 1 out]
                      n198 = call "Serial.vi"("error in (no error)"=w453, "write buffer"=w457, "VISA resource name"=w456) -> ("error out"=w460:errorcluster, "read buffer"=w461:string)  [unwired: 7 in]
                    }
                    frame "Version" {
                      n199 = Concatenate Strings("VR" ("string"), "\r\n" ("write buffer")) -> (w468:string)
                      n200 = property on="Index" class="Ring (strict)"(error in=w464, "DisabledEnum"=T11."Disabled and Grayed Out" ("Disabled")) -> (error out=w463:errorcluster)  [unwired: 1 in, 1 out]
                      n201 = call "Serial.vi"("error in (no error)"=w463, "write buffer"=w468, "VISA resource name"=w466) -> ("error out"=w467:errorcluster, "read buffer"=w462:string)  [unwired: 7 in]
                    }
                  }
                }
                frame "Set" {
                  n202 = To Unsigned Long Integer(number=w491) -> (unsigned 32bit integer=w487:u32)
                  n203 = Number To Decimal String(number=w486) -> (decimal integer string=w485:string)  [unwired: 1 in]
                  n204 = Number To Decimal String(number=w489) -> (decimal integer string=w488:string)  [unwired: 1 in]
                  n205 = case shown="\"Version\"" w479 {
                    tunnel: w478 -> [w499 w503 w507 w511 w515 w519]
                    tunnel: [FALSE TRUE TRUE FALSE FALSE FALSE] -> w476
                    tunnel: [TRUE TRUE TRUE FALSE TRUE FALSE] -> w475
                    tunnel: [FALSE FALSE FALSE TRUE FALSE FALSE] -> w474
                    tunnel: [w499 w503 w507 w511 w515 w519] -> w472
                    frame "Serial Number", Default {
                    }
                    frame "Temperature" {
                    }
                    frame "Unit Adress" {
                    }
                    frame "Calibration" {
                    }
                    frame "Velocity" {
                    }
                    frame "Version" {
                    }
                  }
                  n206 = Number To Decimal String(number=w487) -> (decimal integer string=w490:string)  [unwired: 1 in]
                  n207 = flat-sequence {
                    tunnel: [w522] -> w494
                    tunnel: w471 -> [w522]
                    frame #0 {
                      n208 = Wait (ms)(milliseconds to wait=u32 50) -> ()  [unwired: 1 out]
                    }
                  }
                  n209 = property on="Index" class="Ring (strict)"(error in=w472, "Visible"=w476) -> (error out=w477:errorcluster)  [unwired: 1 in, 1 out]
                  n210 = property on="Value" class="DigNum (strict)"(error in=w477, "Visible"=w475) -> (error out=w473:errorcluster)  [unwired: 1 in, 1 out]
                  n211 = property on="Value 1/2" class="Enum (strict)"(error in=w473, "Visible"=w474) -> (error out=w471:errorcluster)  [unwired: 1 in, 1 out]
                  n212 = case shown="\"Enable Conf. EP=1\"" w479 {
                    tunnel: [w525 w531 w540 w548 w566 "EP=1\r\n" ("write buffer")] -> w480
                    tunnel: w494 -> [w524 w530 w539 w553 w557 w569]
                    tunnel: [w524 w530 w539 w553 w554 w569] -> w493
                    tunnel: w490 -> [w526 w532 w545 _ _ _]
                    tunnel: w488 -> [_ _ _ w549 _ _]
                    tunnel: w487 -> [_ _ _ _ w558 _]
                    tunnel: w485 -> [_ w533 w543 _ _ _]
                    frame "Serial Number", Default {
                      n213 = Concatenate Strings("SN" ("write buffer"), "=" ("string"), w526, "\r\n" ("write buffer")) -> (w525:string)
                    }
                    frame "Temperature" {
                      n214 = Concatenate Strings("TA" ("string"), "[", w533, "]", "=" ("string"), w532, "\r\n" ("write buffer")) -> (w531:string)
                    }
                    frame "Unit Adress" {
                      n215 = Concatenate Strings("UA" ("string"), "[", w543, "]", "=" ("string"), w545, "\r\n" ("write buffer")) -> (w540:string)
                    }
                    frame "Calibration" {
                      n216 = Concatenate Strings("CC" ("string"), "=" ("string"), w549, "\r\n" ("write buffer")) -> (w548:string)
                    }
                    frame "Velocity" {
                      n217 = In Range and Coerce(upper limit=u16 18001, x=w558, lower limit=u16 0) -> (coerced(x)=w564:u32, In Range?=w562:bool)
                      n218 = Not(x=w562) -> (.not. x?=w563:bool)
                      n219 = Select(t=w564, s=w562, f=u16 0) -> (s? t:f=w556:u32)
                      n220 = call "Display Message to User2"("error in (no error)"=w557, "Enable"=w563) -> ("error out"=w554:errorcluster)  [unwired: 8 in, 1 out]
                      n221 = Number To Decimal String(number=w556) -> (decimal integer string=w555:string)  [unwired: 1 in]
                      n222 = Concatenate Strings("VC" ("write buffer"), "=" ("string"), w555, "\r\n" ("write buffer")) -> (w566:string)
                    }
                    frame "Enable Conf. EP=1" {
                    }
                  }
                  n223 = VISA Write(VISA resource name=w492, write buffer=w480, error in (no error)=w493) -> (error out=w495:errorcluster)  [unwired: 2 out]
                  n224 = flat-sequence {
                    tunnel: w495 -> [w520]
                    tunnel: [w520] -> w484
                    frame #0 {
                      n225 = Wait (ms)(milliseconds to wait=u32 50) -> ()  [unwired: 1 out]
                    }
                  }
                  n226 = feedback #1("") -> (w481:string)
                  n227 = Concatenate Strings(w481, w480) -> (w482:string)
                  n228 = feedback-in #1(w482) -> ()
                }
              }
              "read buffer" <- w390
              n229 = Add(x=u32 5, y=w382) -> (x+y=w381:u32)
              n230 = property on="read buffer" class="Str"(error in=w384, "Text.Scroll Position"=w381) -> (error out=w383:errorcluster)  [unwired: 1 in, 1 out]
            }
            event "SetGet": Value Change {
              n231 = event-data() -> ()  [unwired: 1 in, 6 out]
              n232 = property on="Function" class="Enum (strict)"() -> ("Value"=w584:T1)  [unwired: 2 in, 2 out]
              n233 = case shown="\"Version\"" w584 {
                tunnel: w577 -> [w588 w592 w596 w600 w604 w608]
                tunnel: [FALSE TRUE TRUE FALSE FALSE FALSE] -> w582
                tunnel: [TRUE TRUE TRUE FALSE TRUE FALSE] -> w581
                tunnel: [FALSE FALSE FALSE TRUE FALSE FALSE] -> w580
                tunnel: [w588 w592 w596 w600 w604 w608] -> w578
                frame "Serial Number", Default {
                }
                frame "Temperature" {
                }
                frame "Unit Adress" {
                }
                frame "Calibration" {
                }
                frame "Velocity" {
                }
                frame "Version" {
                }
              }
              n234 = property on="Index" class="Ring (strict)"(error in=w578, "Visible"=w582) -> (error out=w583:errorcluster)  [unwired: 1 in, 1 out]
              n235 = property on="Value" class="DigNum (strict)"(error in=w583, "Visible"=w581) -> (error out=w579:errorcluster)  [unwired: 1 in, 1 out]
              n236 = property on="Value 1/2" class="Enum (strict)"(error in=w579, "Visible"=w580) -> (error out=w576:errorcluster)  [unwired: 1 in, 1 out]
            }
            event "Set Param.": Value Change {
              n237 = event-data() -> ()  [unwired: 1 in, 6 out]
              n238 = property on="Serial Status" class="Bool (strict)"(error in=w611) -> (error out=w610:errorcluster, "Value"=w616:bool)  [unwired: 1 in, 1 out]
              n239 = case shown="True" w616 {
                tunnel: w610 -> [w628 w638]
                tunnel: [w627 w633] -> w613
                frame False {
                  n240 = call "Display Message to User4"("error in (no error)"=w628) -> ("error out"=w627:errorcluster)  [unwired: 9 in, 1 out]
                }
                frame True {
                  n241 = property on="Speed control" class="Bool (strict)"(error in=w638, "Visible"=FALSE) -> (error out=w636:errorcluster)  [unwired: 1 in, 1 out]
                  n242 = case shown="47" "Param to Set" {
                    tunnel: [w694 w698 w702] -> w656
                    tunnel: w636 -> [w693 w697 w701]
                    tunnel: [w693 w697 w701] -> w644
                    frame 95, Default {
                      n243 = call <vilib>:"Application Directory.vi"() -> ("Application Directory"=w696:path)
                      n244 = Build Path(base path=w696, name or relative path="data\\Marvin_EBAY_params_RRPAR000017_95_v0.2.txt") -> (appended path=w694:path)
                    }
                    frame 63 {
                      n245 = call <vilib>:"Application Directory.vi"() -> ("Application Directory"=w700:path)
                      n246 = Build Path(base path=w700, name or relative path="data\\Marvin_AHU_params_RRPAR000016_63_v0.2.txt") -> (appended path=w698:path)
                    }
                    frame 47 {
                      n247 = call <vilib>:"Application Directory.vi"() -> ("Application Directory"=w704:path)
                      n248 = Build Path(base path=w704, name or relative path="data\\Marvin_AHU_params_RRPAR000015_47_v0.2.txt") -> (appended path=w702:path)
                    }
                  }
                  n249 = property on="read buffer" class="Str"(error in=w644, "Visible"=TRUE) -> (error out=w640:errorcluster)  [unwired: 1 in, 1 out]
                  n250 = property on="Array" class="Arr (strict)"(error in=w640, "Visible"=FALSE) -> (error out=w639:errorcluster)  [unwired: 1 in, 1 out]
                  n251 = property on="Horizontal Progress Bar" class="Slide (strict)"(error in=w639, "Visible"=TRUE, "Value"=u8 0 ("Horizontal Progress Bar")) -> (error out=w635:errorcluster)  [unwired: 1 in, 1 out]
                  n252 = call <vilib>:"Read Characters From File.vi"("file path (dialog if empty)"=w656) -> ("character string"=w657:string)  [unwired: 5 in, 3 out]
                  n253 = while {
                    shift-right: [w685] -> _
                    shift-left: w657 -> [w686]
                    shift-right: [w681] -> w642
                    shift-left: string[] [] -> [w682]
                    tunnel: w635 -> [w674]
                    tunnel: [w674] -> w654
                    stop <- w687 stop-if-true
                    n254 = Match Pattern(string=w686, regular expression="\r\n") -> (before substring=w683:string, after substring=w685:string, offset past match=w684:i32)  [unwired: 1 in, 1 out]
                    n255 = call <vilib>:"Trim Whitespace.vi"("string"=w683) -> ("trimmed string"=w680:string)  [unwired: 1 in]
                    n256 = Equal?(x=w684, y=-1) -> (x = y?=w687:bool)
                    n257 = To Upper Case(1:w680) -> (0:w678:string)
                    n258 = String Length(string=w678) -> (length=w677:i32)
                    n259 = Greater?(x=w677, y=3) -> (0:w675:bool)
                    n260 = case shown="True" w675 {
                      tunnel: w682 -> [w689 w692]
                      tunnel: [w689 w691] -> w681
                      tunnel: w678 -> [_ w690]
                      frame False {
                      }
                      frame True {
                        n261 = Build Array (concatenate)(w692, w690) -> (w691:string[])
                      }
                    }
                  }
                  n262 = property on="VISA resource name" class="VISAName"(error in=w654) -> (error out=w647:errorcluster, "Value"=w632:refnum<visa-resource-name>)  [unwired: 1 in, 1 out]
                  n263 = Build Array (concatenate)(w642, string[] ["MT", "VR", "SN"] ("array")) -> (w651:string[])
                  n264 = Array Size(array=w651) -> (size(s)=w643:i32)
                  n265 = Bundle By Name(cluster=T12 {"Minimum"=0.0, "Maximum"=0.0, "Increment"=0.0} ("Data Entry Limits"), "Minimum"=0.0, "Maximum"=w643) -> (w649:T12)
                  n266 = property on="Horizontal Progress Bar" class="Slide (strict)"(error in=w647, "Data Range"=w649) -> (error out=w631:errorcluster)  [unwired: 1 in, 1 out]
                  n267 = property on="read buffer" class="Str"(error in=w631) -> (error out=w630:errorcluster, "Text.Scroll Position"=w629:u32)  [unwired: 1 in, 1 out]
                  n268 = for {
                    tunnel: w651 -> [w665] mode=indexing
                    tunnel: w632 -> [w671]
                    tunnel: w630 -> [w670]
                    tunnel: [w662] -> w634
                    tunnel: w629 -> [w661]
                    i -> [w660]
                    n269 = Concatenate Strings(w665, "\r\n" ("string")) -> (w663:string)
                    n270 = VISA Write(VISA resource name=w671, write buffer=w663, error in (no error)=w670) -> (error out=w669:errorcluster)  [unwired: 2 out]
                    n271 = flat-sequence {
                      tunnel: w669 -> [w672]
                      tunnel: [w672] -> w662
                      frame #0 {
                        n272 = Wait (ms)(milliseconds to wait=u32 50) -> ()  [unwired: 1 out]
                      }
                    }
                    n273 = Add(x=w661, y=w660) -> (x+y=w659:u32)
                    n274 = feedback #2("") -> (w667:string)
                    n275 = Concatenate Strings(w667, w663) -> (w668:string)
                    n276 = feedback-in #2(w668) -> ()
                    n277 = property on="read buffer" class="Str"("Value"=w668, "Text.Scroll Position"=w659) -> ()  [unwired: 2 in, 2 out]
                    "Horizontal Progress Bar" <- w660
                  }
                  n278 = VISA Flush I/O Buffer(VISA resource name=w632, error in (no error)=w634) -> (error out=w633:errorcluster)  [unwired: 1 in, 1 out]
                }
              }
              n279 = property on="Serial Monitor" class="Bool (strict)"(error in=w613) -> (error out=w612:errorcluster, "Value"=w614:bool)  [unwired: 1 in, 1 out]
              n280 = case shown="False" w614 {
                tunnel: w612 -> [w625 w626]
                tunnel: [w623 w626] -> w615
                frame False {
                  n281 = property on="read buffer" class="Str"(error in=w625, "Visible"=FALSE) -> (error out=w624:errorcluster)  [unwired: 1 in, 1 out]
                  n282 = property on="Array" class="Arr (strict)"(error in=w624, "Visible"=TRUE) -> (error out=w623:errorcluster)  [unwired: 1 in, 1 out]
                }
                frame True {
                }
              }
            }
            event "Help Button": Value Change {
              n283 = event-data() -> ()  [unwired: 1 in, 6 out]
              n284 = control-ref of="This VI"() -> (w712:refnum<vi>)
              n285 = property class="VI"(reference=w712, error in=w710, "FP:Transparency"=u8 25 ("Front Panel Window:Transparency")) -> (reference out=w706:refnum<vi>, error out=w709:errorcluster)
              n286 = vi-ref "Help.vi"() -> (w716:refnum<vi>)
              n287 = invoke class="VI" method="FP.Open"(reference=w716, error in=w709, "Activate"=TRUE ("Activate?"), "State"=T13."Standard") -> (error out=w715:errorcluster)  [unwired: 1 in, 4 out]
              n288 = call "Help.vi"("error in"=w715) -> ("error out"=w708:errorcluster)  [unwired: 7 in]
              n289 = property class="VI"(reference=w706, error in=w708, "FP:Transparency"=u8 0 ("Front Panel Window:Transparency")) -> (error out=w707:errorcluster)  [unwired: 1 out]
            }
            event "Can Send": Value Change {
              w741 = u8 0 items=["STATUS"=128, "EXTENDED"=2, "RTR"=1, "DATA MSG"=0] ("MSGTYPE")
              w746 = u8 1 items=["Standart flag", "Extern flag"] ("Format")
              w745 = u8 0 items=["Data flag", "Remote flag"] ("Type")
              # "Send"
              n290 = event-data() -> ()  [unwired: 1 in, 6 out]
              n291 = In Range and Coerce(upper limit=u16 18001, x="Motor Speed RPM", lower limit=u16 0) -> (coerced(x)=w727:u16, In Range?=w725:bool)
              n292 = Not(x=w725) -> (.not. x?=w726:bool)
              n293 = Select(t=w727, s=w725, f=u16 0) -> (s? t:f=w729:u16)
              n294 = property on="Unit Adress" class="DigNum (strict)"() -> ("Value"=w723:u8)  [unwired: 2 in, 2 out]
              n295 = Split Number(x=w729) -> (hi(x)=w733:u8, lo(x)=w734:u8)
              n296 = call "Display Message to User"("Enable"=w726) -> ()  [unwired: 9 in, 2 out]
              n297 = case shown="95, Default" w723 {
                tunnel: [u32 417357607 u32 417349415 u32 417345319] -> w724
                frame 95, Default {
                }
                frame 63 {
                }
                frame 47 {
                }
              }
              n298 = case shown="95" w723 {
                tunnel: [w763 w768 w779] -> w739
                tunnel: w734 -> [w762 w767 w778]
                tunnel: w733 -> [w761 w766 w777]
                frame 47, Default {
                  w759 = u8 0 ("element")
                  w760 = u8 1 ("element")
                  n299 = Build Array(w760, w762, w761, w760, w759, w759, w759, w759) -> (w763:u8[])
                }
                frame 63 {
                  w764 = u8 0 ("element")
                  w765 = u8 1 ("element")
                  n300 = Build Array(w765, w767, w766, w765, w764, w764, w764, w764) -> (w768:u8[])
                }
                frame 95 {
                  w775 = u8 0 ("element")
                  n301 = Boolean To (0,1)(Boolean="Speed control") -> (0, 1=w773:i16)
                  n302 = Boolean To (0,1)(Boolean="Motor Over Temp") -> (0, 1=w774:i16)
                  n303 = To Unsigned Byte Integer(number=w773) -> (unsigned 8bit integer=w770:u8)
                  n304 = To Unsigned Byte Integer(number=w774) -> (unsigned 8bit integer=w769:u8)
                  n305 = Build Array(u8 1 ("element"), w778, w777, w770, w769, w775, w775, w775) -> (w779:u8[])
                }
              }
              n306 = Array Size(array=w739) -> (size(s)=w744:i32)
              n307 = call "Array Data to Single Num in Hex.vi"("aDATA"=w739) -> ("Numeric"=→"Data Send":u64)  [unwired: 10 in]
              n308 = To Unsigned Byte Integer(number=w744) -> (unsigned 8bit integer=w742:u8)
              n309 = call "CANAnalData.vi"("ID"=w724, "Data"=w739, "Config"=w737) -> ()  [unwired: 4 in, 5 out]
              n310 = Bundle By Name(cluster=T10 {"ID"=0, "MSGTYPE"=0, "LEN"=0, "aDATA"=[]} ("MsgTX 2"), "ID"=w724, "MSGTYPE"=w741, "LEN"=w742, "aDATA"=w739) -> (w740:T10)
              n311 = Unbundle By Name(w740) -> ("ID"=w754:u32, "LEN"=w755:u8, "aDATA"=w756:u8[])  [unwired: 1 out]
              n312 = property class="Clust (strict)"(reference=w737) -> ("Value"=w753:T8)  [unwired: 1 in, 2 out]
              n313 = Bundle By Name(cluster=T14 {"ID"=0, "TimeStamp"=0, "TimeFlag"=0, "SendType"=0, "RemoteFlag"=0, "ExternFlag"=0, "DataLen"=0, "Data"=[], "Reserved"=[]} ("Send"), "ID"=w754, "RemoteFlag"=w745, "ExternFlag"=w746, "DataLen"=w755, "Data"=w756) -> (w751:T14)
              n314 = Unbundle By Name(w753) -> ("DevType"=w747:T2, "DevIndex"=w748:u32, "CanIndex"=w749:T3)
              n315 = Build Array(w751) -> (w750:T14[])
              n316 = call "VCI_Transmit.vi"("Buffer"=w750, "CANIndex"=w749, "DevIndex"=w748, "DevType"=w747) -> ()  [unwired: 1 in, 7 out]
            }
            event "Graph Button": Value Change {
              w787 = FALSE ("Visible")
              n317 = event-data() -> ()  [unwired: 1 in, 6 out]
              n318 = Not(x="Graph Button") -> (.not. x?=w802:bool)
              n319 = property on="Array" class="Arr (strict)"(error in=w798, "Visible"=w802) -> (error out=w801:errorcluster)  [unwired: 1 in, 1 out]
              n320 = property on="Waveform Chart" class="WFChart (strict)"(error in=w801, "Visible"="Graph Button") -> (error out=w797:errorcluster)  [unwired: 1 in, 1 out]
              n321 = property on="Serial Monitor" class="Bool (strict)"(error in=w797) -> (error out=w799:errorcluster, "Value"=w800:bool)  [unwired: 1 in, 1 out]
              n322 = case shown="True" w800 {
                tunnel: w799 -> [w810 w813]
                tunnel: [w808 w811] -> w785
                frame False {
                  n323 = property on="read buffer" class="Str"(error in=w810, "Visible"=FALSE) -> (error out=w808:errorcluster)  [unwired: 1 in, 1 out]
                }
                frame True {
                  n324 = property on="read buffer" class="Str"(error in=w813, "Visible"=TRUE) -> (error out=w815:errorcluster)  [unwired: 1 in, 1 out]
                  n325 = property on="Array" class="Arr (strict)"(error in=w815, "Visible"=FALSE) -> (error out=w811:errorcluster)  [unwired: 1 in, 1 out]
                }
              }
              n326 = property on="Serial Monitor" class="Bool (strict)"(error in=w785, "Value"=FALSE ("Serial Monitor")) -> (error out=w783:errorcluster)  [unwired: 1 in, 1 out]
              n327 = property on="Index" class="Ring (strict)"(error in=w783, "Visible"=w787) -> (error out=w794:errorcluster)  [unwired: 1 in, 1 out]
              n328 = property on="Value 1/2" class="Enum (strict)"(error in=w794, "Visible"=w787) -> (error out=w793:errorcluster)  [unwired: 1 in, 1 out]
              n329 = property on="Value" class="DigNum (strict)"(error in=w793, "Visible"=w787) -> (error out=w792:errorcluster)  [unwired: 1 in, 1 out]
              n330 = property on="SetGet" class="Enum (strict)"(error in=w792, "Visible"=w787) -> (error out=w791:errorcluster)  [unwired: 1 in, 1 out]
              n331 = property on="Serial Send" class="Bool"(error in=w791, "Visible"=w787) -> (error out=w789:errorcluster)  [unwired: 1 in, 1 out]
              n332 = property on="Clear Monitor" class="Bool"(error in=w789, "Visible"=w787) -> (error out=w788:errorcluster)  [unwired: 1 in, 1 out]
              n333 = property on="Function" class="Enum (strict)"(error in=w788, "Visible"=w787) -> (error out=w790:errorcluster)  [unwired: 1 in, 1 out]
              n334 = property on="Index" class="Ring (strict)"(error in=w790, "Visible"=w787) -> (error out=w795:errorcluster)  [unwired: 1 in, 1 out]
              n335 = property on="read buffer" class="Str"(error in=w795, "Visible"=w787) -> (error out=w786:errorcluster)  [unwired: 1 in, 1 out]
            }
            event "Serial Com": Value Change {
              n336 = event-data() -> ()  [unwired: 1 in, 6 out]
              n337 = property on="Serial Com" class="Bool"(error in=w820, "Visible"=FALSE) -> (error out=w819:errorcluster)  [unwired: 1 in, 1 out]
              n338 = property on="VISA resource name" class="VISAName"(error in=w819, "Visible"=TRUE) -> (error out=w817:errorcluster)  [unwired: 1 in, 1 out]
            }
            event "VISA resource name": Value Change {
              n339 = event-data() -> ()  [unwired: 1 in, 1 out]
              n340 = control-ref of="This VI"() -> (w826:refnum<vi>)
              n341 = call "Serial InitMarvin.vi"("error in (no error)"=w833, "VI reference (current VI)"=w826, "VISA Refnum in"="VISA resource name") -> ("error out"=w842:errorcluster, "Boolean"=w829:bool)  [unwired: 7 in]
              n342 = property on="Serial Status" class="Bool (strict)"(error in=w842, "Value"=w829) -> (error out=w836:errorcluster)  [unwired: 1 in, 1 out]
              n343 = property on="VISA resource name" class="VISAName"(error in=w836, "Visible"=FALSE) -> (error out=w835:errorcluster)  [unwired: 1 in, 1 out]
              n344 = property on="Serial Com" class="Bool"(error in=w835, "Visible"=TRUE) -> (error out=w832:errorcluster)  [unwired: 1 in, 1 out]
              n345 = call <vilib>:"Clear Errors.vi"("error in (no error)"=w832) -> ("error out"=w831:errorcluster)  [unwired: 5 in, 1 out]
              n346 = case shown="True" w829 {
                tunnel: w831 -> [w843 w846]
                tunnel: [w843 w845] -> w830
                tunnel: "VISA resource name" -> [_ w844]
                frame False {
                }
                frame True {
                  n347 = VISA Flush I/O Buffer(VISA resource name=w844, error in (no error)=w846) -> (error out=w845:errorcluster)  [unwired: 1 in, 1 out]
                }
              }
            }
            event "Stop": Value Change {
              n348 = event-data() -> ()  [unwired: 1 in, 6 out]
              n349 = Flush Queue(queue=w852, error in (no error)=w851) -> (queue out=w850:refnum<queue>, error out=w849:errorcluster)  [unwired: 1 out]
              n350 = Release Queue(queue=w850, error in (no error)=w849) -> (error out=w848:errorcluster)  [unwired: 1 in, 2 out]
            }
            event "Refresh Button": Value Change {
              n351 = event-data() -> ()  [unwired: 1 in, 6 out]
              n352 = Release Queue(queue=w858, error in (no error)=w859) -> (error out=w857:errorcluster)  [unwired: 1 in, 2 out]
            }
          }
          n353 = Unbundle By Name(w225) -> ("status"=w231:bool)
          n354 = Or(x=w231, y=w223) -> (x .or. y?=w230:bool)
        }
      }
      frame "Stop" {
        n355 = Release Queue(queue=w866, error in (no error)=w868) -> (error out=w867:errorcluster)  [unwired: 1 in, 2 out]
        n356 = flat-sequence {
          tunnel: w865 -> [w877]
          tunnel: [TRUE ("Stop")] -> w864
          frame #0 {
            w876 = u8[] [1, 0, 0, 0, 0, 0, 0, 0] ("Data 2")
            w879 = u8 0 items=["STATUS"=128, "EXTENDED"=2, "RTR"=1, "DATA MSG"=0] ("MSGTYPE")
            w884 = u8 1 items=["Standart flag", "Extern flag"] ("Format")
            w883 = u8 0 items=["Data flag", "Remote flag"] ("Type")
            n357 = property on="Serial Status" class="Bool (strict)"() -> ("Value"=w869:bool)  [unwired: 2 in, 2 out]
            n358 = property on="Unit Adress" class="DigNum (strict)"() -> ("Value"=w871:u8)  [unwired: 2 in, 2 out]
            n359 = case shown="True" w869 {
              frame False {
              }
              frame True {
                n360 = property on="VISA resource name" class="VISAName"() -> ("Value"=w895:refnum<visa-resource-name>)  [unwired: 2 in, 2 out]
                n361 = VISA Close(VISA resource name=w895) -> ()  [unwired: 1 in, 1 out]
              }
            }
            n362 = case shown="95, Default" w871 {
              tunnel: [u32 417357607 u32 417349415 u32 417345319] -> w870
              frame 95, Default {
              }
              frame 63 {
              }
              frame 47 {
              }
            }
            n363 = property on="Graph Button" class="Bool (strict)"("Value"=FALSE ("Graph Button")) -> ()  [unwired: 2 in, 2 out]
            n364 = Array Size(array=w876) -> (size(s)=w882:i32)
            n365 = To Unsigned Byte Integer(number=w882) -> (unsigned 8bit integer=w880:u8)
            n366 = property on="Waveform Chart" class="WFChart (strict)"("Visible"=FALSE, "Value"=dbl[] [] ("Waveform Chart")) -> ()  [unwired: 2 in, 2 out]
            n367 = Bundle By Name(cluster=T10 {"ID"=0, "MSGTYPE"=0, "LEN"=0, "aDATA"=[]} ("MsgTX 2"), "ID"=w870, "MSGTYPE"=w879, "LEN"=w880, "aDATA"=w876) -> (w878:T10)
            n368 = call "CANAnalData.vi"("ID"=w870, "Data"=w876, "Config"=w877) -> ()  [unwired: 4 in, 5 out]
            n369 = call "Array Data to Single Num in Hex.vi"("aDATA"=w876) -> ("Numeric"=w875:u64)  [unwired: 10 in]
            n370 = property on="Data Send" class="DigNum (strict)"("Value"=w875) -> ()  [unwired: 2 in, 2 out]
            n371 = Unbundle By Name(w878) -> ("ID"=w892:u32, "LEN"=w893:u8, "aDATA"=w894:u8[])  [unwired: 1 out]
            n372 = property class="Clust (strict)"(reference=w877) -> ("Value"=w891:T8)  [unwired: 1 in, 2 out]
            n373 = Bundle By Name(cluster=T14 {"ID"=0, "TimeStamp"=0, "TimeFlag"=0, "SendType"=0, "RemoteFlag"=0, "ExternFlag"=0, "DataLen"=0, "Data"=[], "Reserved"=[]} ("Send"), "ID"=w892, "RemoteFlag"=w883, "ExternFlag"=w884, "DataLen"=w893, "Data"=w894) -> (w889:T14)
            n374 = Unbundle By Name(w891) -> ("DevType"=w885:T2, "DevIndex"=w886:u32, "CanIndex"=w887:T3)
            n375 = Build Array(w889) -> (w888:T14[])
            n376 = call "VCI_Transmit.vi"("Buffer"=w888, "CANIndex"=w887, "DevIndex"=w886, "DevType"=w885) -> ()  [unwired: 1 in, 7 out]
          }
          frame #1 {
          }
        }
      }
    }
  }
